vi "DSF.Engine.Plugin.Get Transfer Configuration.vi"(8 "error in (no error)":errorcluster, 11 "Plugin in":refnum<class "Plugin.lvclass">) -> (0 "error out":errorcluster, 2 "Transfer Configuration":refnum<class "DSF.Shared.Configuration.Transfer.lvclass">, 3 "Plugin out":refnum<class "Plugin.lvclass">)   [LabVIEW 2016, in "DSF.Engine.lvlib" / "Plugin.lvclass"]
uses:
  Plugin.lvclass
  Shared/Classes/Transfer/DSF.Shared.Configuration.Transfer.lvclass
  Plugin.lvclass/Plugin.ctl
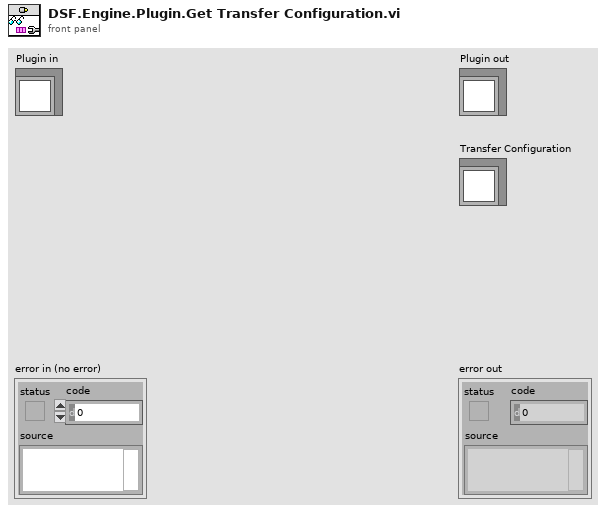
[diagram p1: front panel]
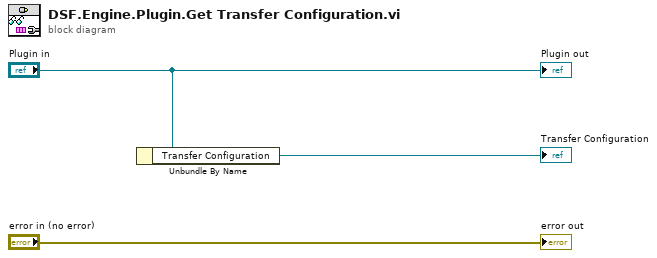
[diagram p0: block diagram]
diagram:
  n1 = Unbundle By Name("Plugin in") -> ("Transfer Configuration"=→"Transfer Configuration":refnum<class "DSF.Shared.Configuration.Transfer.lvclass">)
  "error out" <- "error in (no error)"
  "Plugin out" <- "Plugin in"
